vi "Party Time Drive Too - Xbox.vi"(11 "Controller Values":T1) -> (2 "Right Setpoint":dbl, 3 "Left Setpoint":dbl)   [LabVIEW 2018]
uses:
  Controller Values.ctl
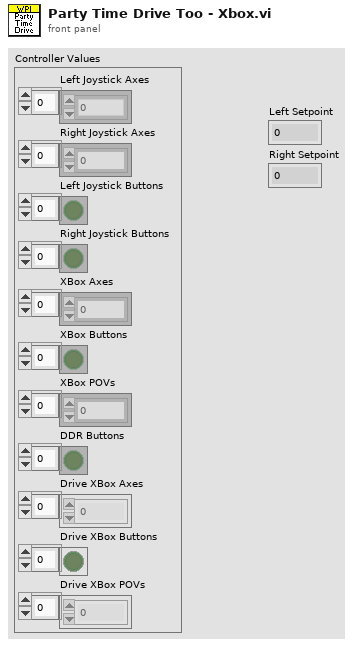
[diagram p1: front panel]
types:
  T1 = typedef "Controller Values.ctl" = cluster{"Left Joystick Axes ":dbl[], "Right Joystick Axes":dbl[], "Left Joystick Buttons":bool[], "Right Joystick Buttons":bool[], "XBox Axes":dbl[], "XBox Buttons":bool[], "XBox POVs":i16[], "DDR Buttons":bool[], "Drive XBox Axes":dbl[], "Drive XBox Buttons":bool[], "Drive XBox POVs":i16[]}
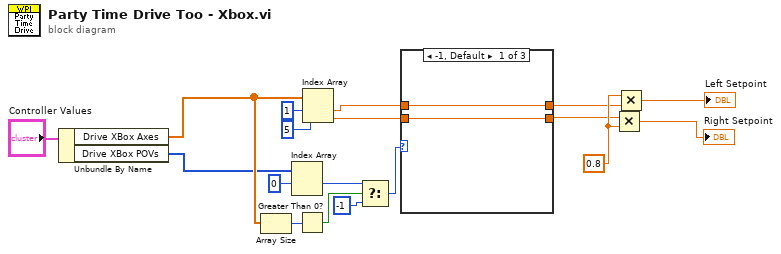
[diagram p0: block diagram]
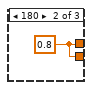
[diagram p2: hidden frame]
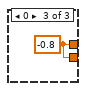
[diagram p3: hidden frame]
diagram:
  w10 = 0.8 ("y")
  n1 = Unbundle By Name("Controller Values") -> ("Drive XBox Axes"=w2:dbl[], "Drive XBox POVs"=w1:i16[])
  n2 = Array Size(array=w2) -> (size(s)=w8:i32)
  n3 = Index Array(array=w1, index #1=0 ("index")) -> (element #1=w11:i16)  [unwired: 1 in, 1 out]
  n4 = Greater Than 0?(x=w8) -> (x > 0?=w7:bool)
  n5 = Index Array(array=w2, index #1=1 ("index"), index #2=5 ("index")) -> (element #1=w16:dbl, element #2=w15:dbl)
  n6 = Select(t=w11, s=w7, f=i16 -1) -> (s? t:f=w12:i16)
  n7 = case shown="-1, Default" w12 {
    tunnel: w16 -> [w20 _ _]
    tunnel: [w20 w21 w22] -> w6
    tunnel: w15 -> [w19 _ _]
    tunnel: [w19 w21 w22] -> w5
    frame -1, Default {
    }
    frame 180 {
      w21 = 0.8 ("upper limit")
    }
    frame 0 {
      w22 = -0.8 ("upper limit")
    }
  }
  n8 = Multiply(x=w5, y=w10) -> (x*y=→"Right Setpoint":dbl)
  n9 = Multiply(x=w10, y=w6) -> (x*y=→"Left Setpoint":dbl)
